vi "make_rep_trial_folder_str.vi"(6 "trial":i32, 8 "rep":i32) -> (5 "folder string":string)   [LabVIEW 2015]
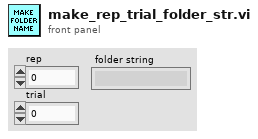
[diagram p1: front panel]
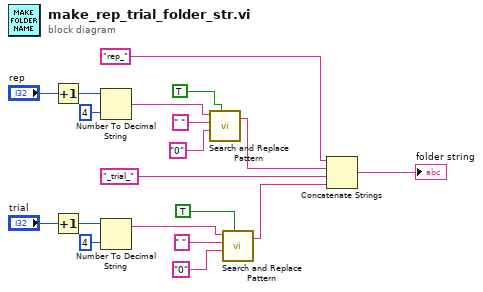
[diagram p0: block diagram]
diagram:
  n1 = Increment(x="rep") -> (x+1=w2:i32)
  n2 = Increment(x="trial") -> (x+1=w5:i32)
  n3 = Number To Decimal String(number=w2, width (-)=i16 4) -> (decimal integer string=w7:string)
  n4 = Number To Decimal String(number=w5, width (-)=i16 4) -> (decimal integer string=w11:string)
  n5 = call <vilib>:"Search and Replace Pattern.vi"("string"=w7, "regular expression (\"\")"=" " ("regular expression (\"\")"), "replace string (\"\")"="0" ("replace string (\"\")"), "replace all? (F)"=TRUE) -> ("result string"=w6:string)  [unwired: 1 in, 1 out]
  n6 = call <vilib>:"Search and Replace Pattern.vi"("string"=w11, "regular expression (\"\")"=" " ("regular expression (\"\")"), "replace string (\"\")"="0" ("replace string (\"\")"), "replace all? (F)"=TRUE) -> ("result string"=w12:string)  [unwired: 1 in, 1 out]
  n7 = Concatenate Strings("rep_", w6, "_trial_", w12) -> (→"folder string":string)
